vi "Send UI Reference.vi"(8 "error in (no error)":errorcluster, 11 "Stage Controller StepMotor in":refnum<class "Stage Controller StepMotor.lvclass">) -> (0 "error out":errorcluster, 3 "Stage Controller StepMotor out":refnum<class "Stage Controller StepMotor.lvclass">)   [LabVIEW 2020, in "Stage.lvlib" / "Stage Controller StepMotor.lvlib" / "Stage Controller StepMotor.lvclass"]
uses:
  Stage Controller StepMotor.lvclass
  C:/Program Files/National Instruments/LabVIEW 2020/vi.lib/ActorFramework/Actor/Actor.lvclass
  <vilib>/ActorFramework/Actor/Actor.lvclass/Actor.ctl
  Stage Controller StepMotor.lvclass/Stage Controller StepMotor.ctl
  Device/Device Messages/SendPanelUIReference Msg/SendPanelUIReference Msg.lvclass/SendPanelUIReference Msg.ctl
  <vilib>/ActorFramework/Message Enqueuer/Message Enqueuer.lvclass/Message Enqueuer.ctl
  <vilib>/ActorFramework/Message Enqueuer/Enqueue.vi
  Device/Device Messages/SendPanelUIReference Msg/SendPanelUIReference Msg.lvclass
  C:/Program Files/National Instruments/LabVIEW 2020/vi.lib/ActorFramework/Message/Message.lvclass
  <vilib>/ActorFramework/Message Priority Queue/Priority Enqueue.vi
  <vilib>/ActorFramework/Actor/Actor.lvclass
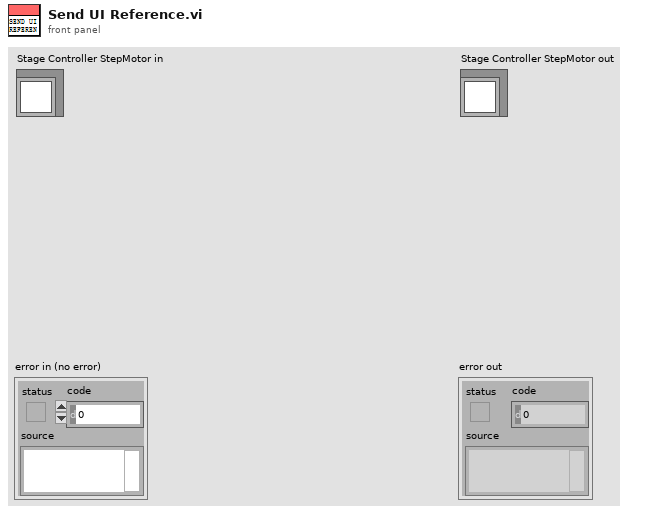
[diagram p1: front panel]
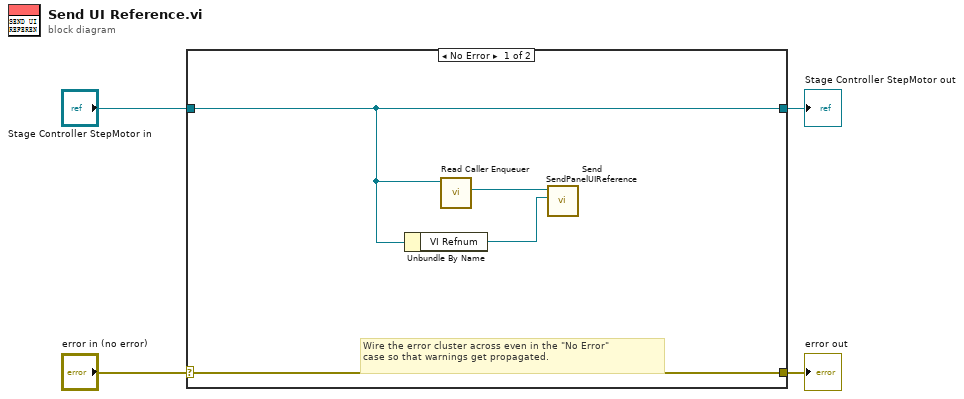
[diagram p0: block diagram]
diagram:
  n1 = case shown="No Error" "error in (no error)" {
    selector: "error in (no error)" -> [w8 w10]
    tunnel: [w8 w10] -> w3
    tunnel: [w5 w9] -> w1
    tunnel: "Stage Controller StepMotor in" -> [w5 w9]
    frame No Error {
      # "Wire the error cluster across even in the \"No Error\"\ncase so that warnings get propagated."
      n2 = Unbundle By Name(w5) -> ("VI Refnum"=w6:refnum<vi>)
      n3 = call <vilib>:"Read Caller Enqueuer.vi"("Actor"=w5) -> ("Caller Enqueuer"=w7:refnum<class "Message Enqueuer.lvclass">)  [unwired: 10 in]
      n4 = call "Send SendPanelUIReference.vi"("VI Refnum"=w6, "Message Enqueuer"=w7) -> ()  [unwired: 8 in, 2 out]
    }
    frame Error {
    }
  }
  "error out" <- w3
  "Stage Controller StepMotor out" <- w1
